vi "JAUS Message Sorter.vi"() -> ()   [LabVIEW 2009]
uses:
  Support Files/JUDP Read Queue Element.ctl
  Support Files/Address.ctl
  Support Files/Simple Services Receive Triggers.ctl
  Support Files/Complex Services Statechart/Complex Services Queue Element.ctl
  Support Files/Complex Services Statechart/ComplexServices.lvsc/Trigger.ctl
  cRIO/Functional Global Variables/Actions for FG's.ctl
  Support Files/Complex Services Statechart/ComplexServices.lvsc
panel:
  out "Numeric":u16 format="%.0x"
  out "HB":bool
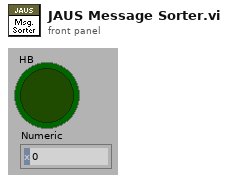
[diagram p1: front panel]
types:
  T1 = typedef "Complex Services Queue Element.ctl" = cluster{"Trigger":T2, "Payload":string, "Sender ID":T3}
  T2 = typedef "ComplexServices.lvsc/Trigger.ctl" = enum16{"NULL", "ReceiveRequestControl", "ReceiveQueryControl", "ReceiveShutdown", "ReceiveQueryStatus", "ReceiveStandby", "ReceiveResume", "Timeout", "Initialized", "Failure", "ReceiveQueryLocalPose", "ReceiveSetLocalPose", "ReceiveQueryElementList", "ReceiveQueryElementCount", "ReceiveSetElement", "ReceiveExecuteList", "ReceiveQueryTravelSpeed", "ReceiveQueryLocalWaypoint", "ReceiveQueryActiveElement"}
  T3 = typedef "Address.ctl" = cluster{"Subsystem Id":u16, "Node Id":u8, "Component Id":u8}
  T4 = typedef "Simple Services Receive Triggers.ctl" = enum16{"NULL", "ReceiveQueryIdentification", "ReceiveQueryServices", "ReceiveQueryVelocityState"}
  T5 = cluster{"Trigger":T4, "Payload":string, "Sender ID":T3}
  T6 = typedef "JUDP Read Queue Element.ctl" = cluster{"Payload":string, "Sender ID":T3, "Command Code":u16}
  T7 = typedef "Actions for FG's.ctl" = enum16{"Read", "Write"}
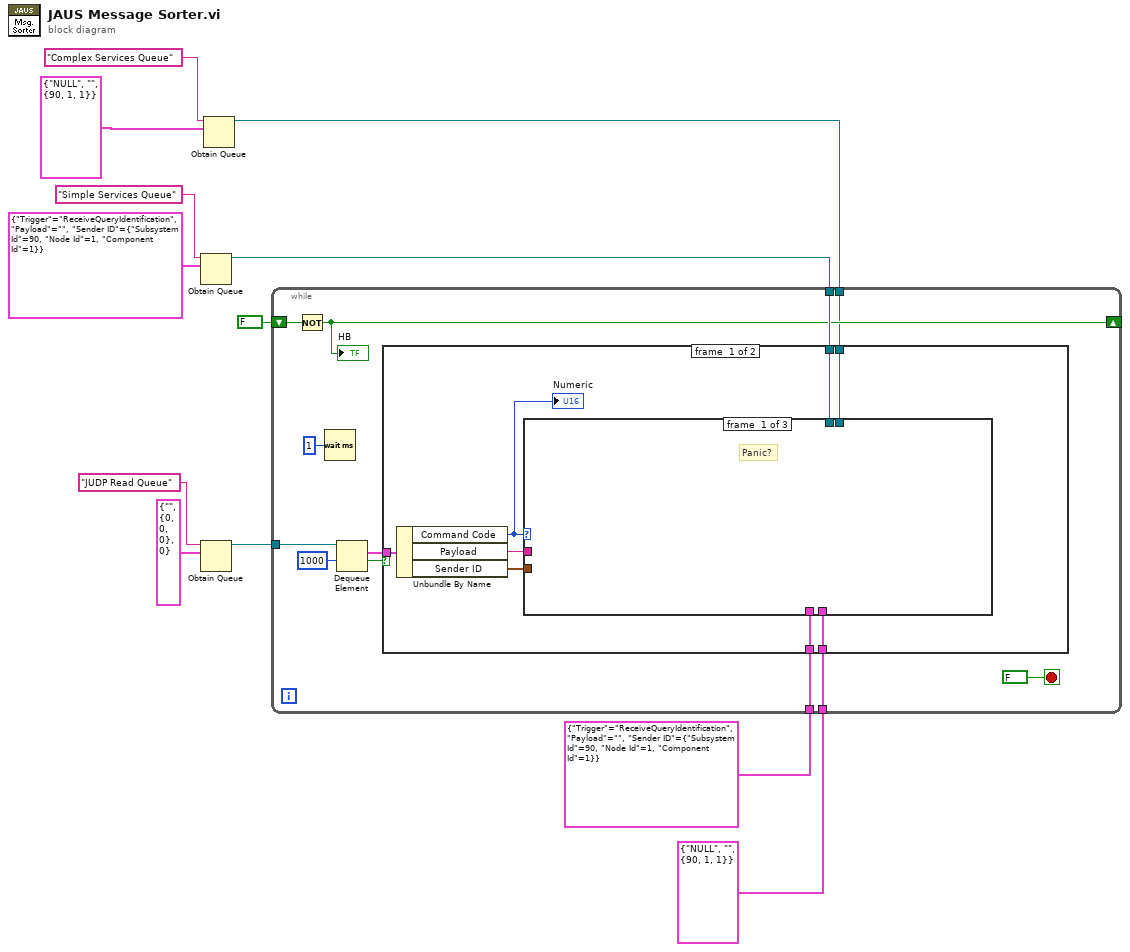
[diagram p0: block diagram]
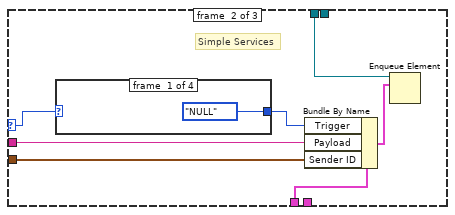
[diagram p2: hidden frame]
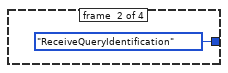
[diagram p3: hidden frame]
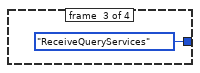
[diagram p4: hidden frame]
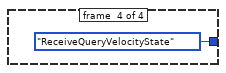
[diagram p5: hidden frame]
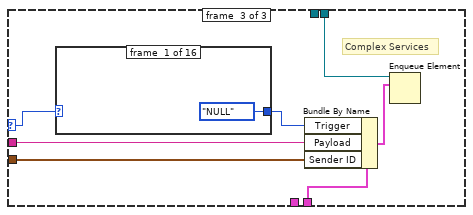
[diagram p6: hidden frame]
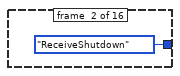
[diagram p7: hidden frame]
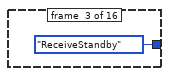
[diagram p8: hidden frame]
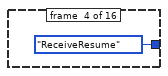
[diagram p9: hidden frame]
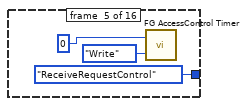
[diagram p10: hidden frame]
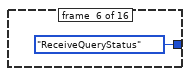
[diagram p11: hidden frame]
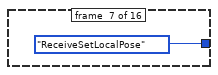
[diagram p12: hidden frame]
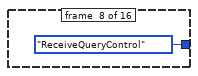
[diagram p13: hidden frame]
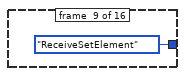
[diagram p14: hidden frame]
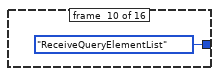
[diagram p15: hidden frame]
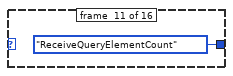
[diagram p16: hidden frame]
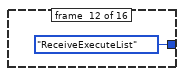
[diagram p17: hidden frame]
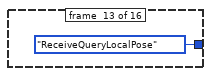
[diagram p18: hidden frame]
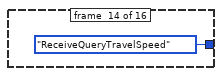
[diagram p19: hidden frame]
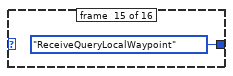
[diagram p20: hidden frame]
diagram:
  n1 = Obtain Queue(name (unnamed)="Simple Services Queue", element data type=T5 {"Trigger"=enum."ReceiveQueryIdentification", "Payload"="", "Sender ID"={"Subsystem Id"=90, "Node Id"=1, "Component Id"=1}} ("Receive FSM Queue Element")) -> (queue out=w7:refnum<queue>)  [unwired: 3 in, 2 out]
  n2 = Obtain Queue(name (unnamed)="JUDP Read Queue", element data type=T6 {"Payload"="", "Sender ID"={"Subsystem Id"=0, "Node Id"=0, "Component Id"=0}, "Command Code"=0} ("Receive FSM Queue Element")) -> (queue out=w10:refnum<queue>)  [unwired: 3 in, 2 out]
  n3 = Obtain Queue(name (unnamed)="Complex Services Queue", element data type=T1 {"Trigger"=enum."NULL", "Payload"="", "Sender ID"={"Subsystem Id"=90, "Node Id"=1, "Component Id"=1}} ("Queue Element")) -> (queue out=w3:refnum<queue>)  [unwired: 3 in, 2 out]
  n4 = while {
    tunnel: w10 -> [w24]
    tunnel: w7 -> [w20]
    tunnel: T5 {"Trigger"=enum."ReceiveQueryIdentification", "Payload"="", "Sender ID"={"Subsystem Id"=90, "Node Id"=1, "Component Id"=1}} ("Receive FSM Queue Element") -> [w19]
    shift-right: [w16] -> _
    shift-left: FALSE ("timed out?") -> [w17]
    tunnel: w3 -> [w14]
    tunnel: T1 {"Trigger"=enum."NULL", "Payload"="", "Sender ID"={"Subsystem Id"=90, "Node Id"=1, "Component Id"=1}} ("Queue Element") -> [w13]
    stop <- FALSE stop-if-true
    n5 = Not(x=w17) -> (.not. x?=w16:bool)
    "HB" <- w16
    n6 = Wait (ms)(milliseconds to wait=u32 1) -> ()  [unwired: 1 out]
    n7 = Dequeue Element(queue=w24, timeout in ms (-1)=1000) -> (element=w22:T6, timed out?=w21:bool)  [unwired: 1 in, 2 out]
    n8 = case shown="False" w21 {
      tunnel: w22 -> [w32 _]
      tunnel: w20 -> [w29 _]
      tunnel: w19 -> [w28 _]
      tunnel: w14 -> [w27 _]
      tunnel: w13 -> [w26 _]
      frame #0 {
        n9 = Unbundle By Name(w32) -> ("Command Code"=w25:u16, "Payload"=w31:string, "Sender ID"=w30:T3)
        "Numeric" <- w25
        n10 = case shown="2..4, D, 403, 41A, 41E, 2002, 200D, 2403, 240A, 240D, 241B, 241C, 241E" w25 {
          selector: w25 -> [_ w39 w44]
          tunnel: w31 -> [_ w37 w47]
          tunnel: w30 -> [_ w36 w46]
          tunnel: w29 -> [_ w34 _]
          tunnel: w28 -> [_ w33 _]
          tunnel: w27 -> [_ _ w50]
          tunnel: w26 -> [_ _ w49]
          frame #0 {
            # "Panic?"
          }
          frame #1 {
            # "Simple Services"
            n11 = case shown="2404" w39 {
              tunnel: [Simple_Services_Receive_Triggers."NULL" ("Trigger") Simple_Services_Receive_Triggers."ReceiveQueryIdentification" ("Trigger") Simple_Services_Receive_Triggers."ReceiveQueryServices" ("Trigger") Simple_Services_Receive_Triggers."ReceiveQueryVelocityState" ("Trigger")] -> w38
              frame #0 {
              }
              frame #1 {
              }
              frame #2 {
              }
              frame #3 {
              }
            }
            n12 = Bundle By Name(cluster=w33, "Trigger"=w38, "Payload"=w37, "Sender ID"=w36) -> (w35:T5)
            n13 = Enqueue Element(queue=w34, element=w35) -> ()  [unwired: 2 in, 3 out]
          }
          frame #2 {
            # "Complex Services"
            n14 = case shown="403" w44 {
              tunnel: [Trigger."NULL" ("Trigger") Trigger."ReceiveShutdown" ("Trigger") Trigger."ReceiveStandby" ("Trigger") Trigger."ReceiveResume" ("Trigger") Trigger."ReceiveRequestControl" ("Trigger") Trigger."ReceiveQueryStatus" ("Trigger") Trigger."ReceiveSetLocalPose" ("Trigger") Trigger."ReceiveQueryControl" ("Trigger") Trigger."ReceiveSetElement" ("Trigger") Trigger."ReceiveQueryElementList" ("Trigger") Trigger."ReceiveQueryElementCount" ("Trigger") Trigger."ReceiveExecuteList" ("Trigger") Trigger."ReceiveQueryLocalPose" ("Trigger") Trigger."ReceiveQueryTravelSpeed" ("Trigger") Trigger."ReceiveQueryLocalWaypoint" ("Trigger") Trigger."ReceiveQueryActiveElement" ("Trigger")] -> w45
              frame #0 {
              }
              frame #1 {
              }
              frame #2 {
              }
              frame #3 {
              }
              frame #4 {
                n15 = call "FG AccessControl Timer.vi"("FG Action (Read)"=Actions_for_FG's."Write", "Count in"=0) -> ()  [unwired: 1 out]
              }
              frame #5 {
              }
              frame #6 {
              }
              frame #7 {
              }
              frame #8 {
              }
              frame #9 {
              }
              frame #10 {
              }
              frame #11 {
              }
              frame #12 {
              }
              frame #13 {
              }
              frame #14 {
              }
              frame #15 {
              }
            }
            n16 = Bundle By Name(cluster=w49, "Trigger"=w45, "Payload"=w47, "Sender ID"=w46) -> (w48:T1)
            n17 = Enqueue Element(queue=w50, element=w48) -> ()  [unwired: 2 in, 3 out]
          }
        }
      }
      frame #1 {
      }
    }
  }
